vi "BT_address_string.vi"(3 "string":string) -> (0 "hex integer string":string[](array[string]), 1 "output array":u8[](array[numeric]))   [LabVIEW 2014]
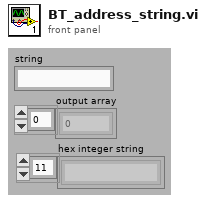
[diagram p1: front panel]
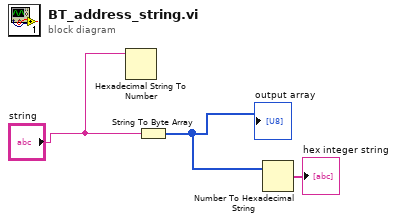
[diagram p0: block diagram]
diagram:
  n1 = Hexadecimal String To Number(string="string") -> ()  [unwired: 2 in, 2 out]
  n2 = String To Byte Array(string="string") -> (unsigned byte array=w2:u8[])
  "output array" <- w2
  n3 = Number To Hexadecimal String(2:w2) -> (0:→"hex integer string":string[])  [unwired: 1 in]
